vi "RTS Macro Power Filter.vi"(0 "Filtered Time":dbl[](array[numeric]), 5 "Filtered Power Factor":dbl[](array[numeric]), 7 "Filtered Power Data":dbl[](array[numeric]), 9 "Filtered Wh Data":dbl[](array[numeric]), 11 "Error In":errorcluster, 12 "Top Compressor Range Data":dbl) -> (4 "Time Output":dbl[](array[numeric]), 6 "Power Output":dbl[](array[numeric]), 10 "Power Factor Output":dbl[](array[numeric]), 15 "Error Out":errorcluster)   [LabVIEW 2016]
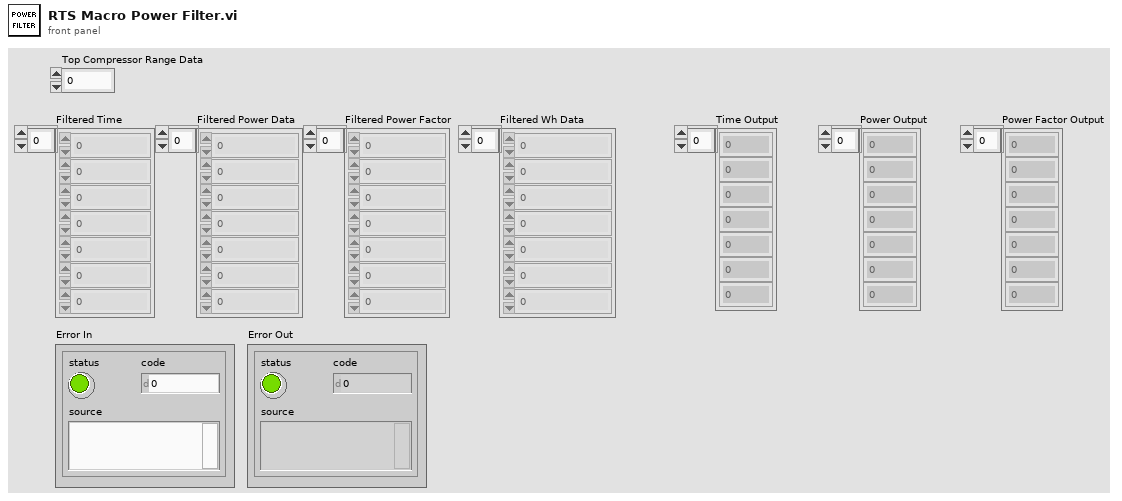
[diagram p1: front panel]
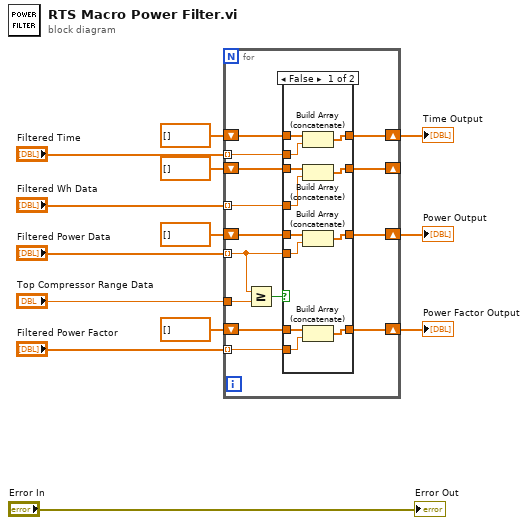
[diagram p0: block diagram]
diagram:
  n1 = for {
    tunnel: "Filtered Power Data" -> [w23] mode=indexing
    tunnel: "Top Compressor Range Data" -> [w27]
    shift-right: [w24] -> w12
    shift-left: dbl[] [] -> [w25]
    tunnel: "Filtered Time" -> [w20] mode=indexing
    shift-right: [w21] -> w11
    shift-left: dbl[] [] -> [w22]
    shift-right: [w18] -> _
    shift-left: dbl[] [] -> [w19]
    tunnel: "Filtered Wh Data" -> [w17] mode=indexing
    shift-right: [w15] -> w13
    shift-left: dbl[] [] -> [w16]
    tunnel: "Filtered Power Factor" -> [w14] mode=indexing
    n2 = Greater Or Equal?(x=w23, y=w27) -> (x >= y?=w26:bool)
    n3 = case shown="False" w26 {
      tunnel: w25 -> [w39 w43]
      tunnel: [w38 w43] -> w24
      tunnel: w23 -> [w37 _]
      tunnel: w22 -> [w36 w42]
      tunnel: [w35 w42] -> w21
      tunnel: w20 -> [w34 _]
      tunnel: w19 -> [w33 w41]
      tunnel: [w32 w41] -> w18
      tunnel: w17 -> [w31 _]
      tunnel: w16 -> [w30 w40]
      tunnel: [w29 w40] -> w15
      tunnel: w14 -> [w28 _]
      frame False {
        n4 = Build Array (concatenate)(w36, w34) -> (w35:dbl[])
        n5 = Build Array (concatenate)(w33, w31) -> (w32:dbl[])
        n6 = Build Array (concatenate)(w39, w37) -> (w38:dbl[])
        n7 = Build Array (concatenate)(w30, w28) -> (w29:dbl[])
      }
      frame True {
      }
    }
  }
  "Power Factor Output" <- w13
  "Power Output" <- w12
  "Time Output" <- w11
  "Error Out" <- "Error In"
